vi "New Project.vi"(8 "error in (no error)":errorcluster, 11 "Editor.lvclass in":refnum<data-value>) -> (0 "error out":errorcluster, 2 "Cancelled":bool caption="cancelled", 3 "Editor.lvclass out":refnum<data-value>)   [LabVIEW 2015, in "Editor.lvclass"]
uses:
  Editor.lvclass
  Project.lvclass
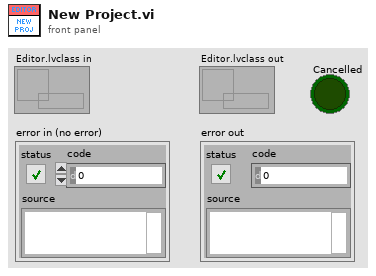
[diagram p1: front panel]
types:
  T1 = enum16{"Left Button", "Center Button", "Right Button", "Window Close"}
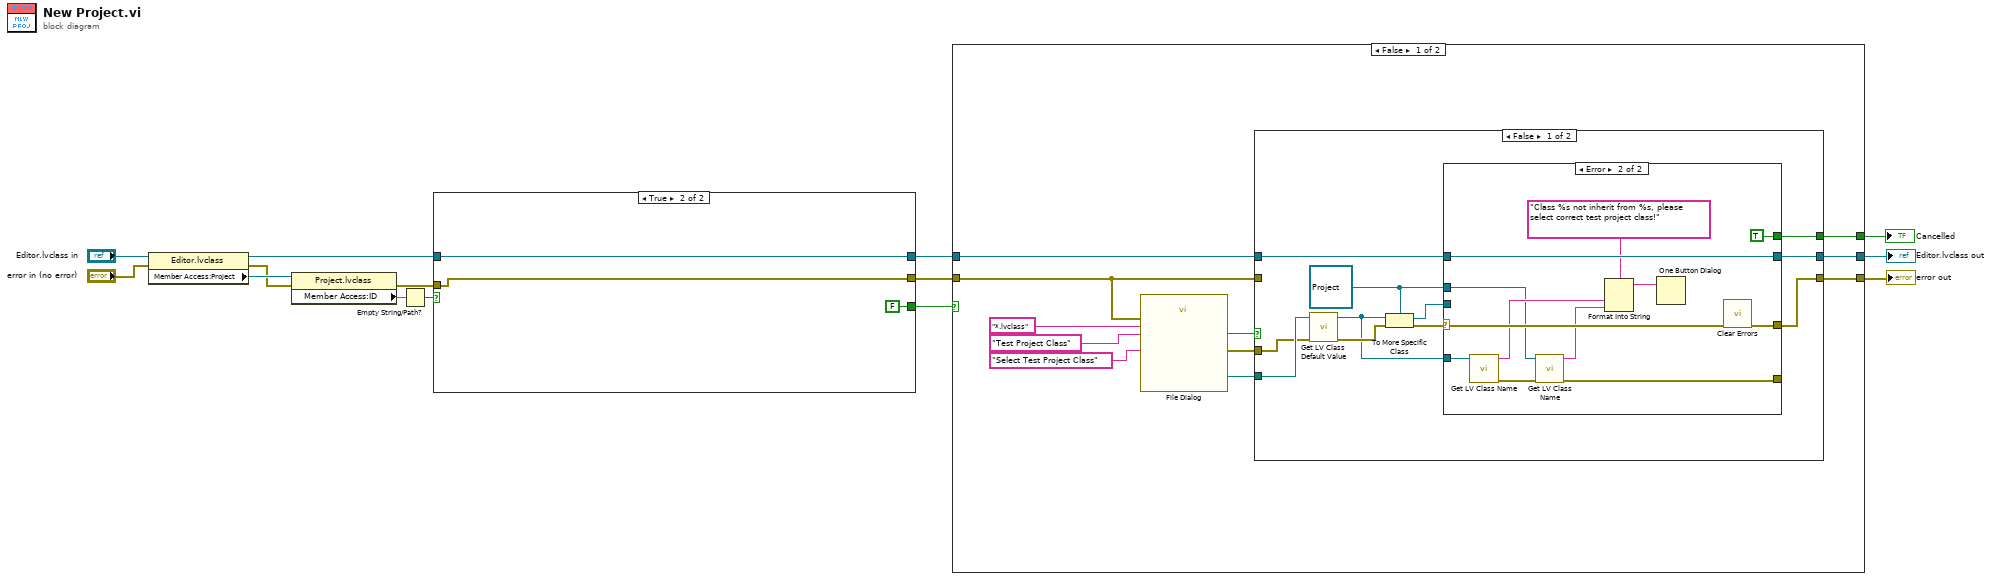
[diagram p0: block diagram]
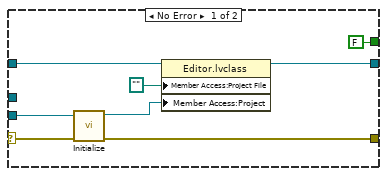
[diagram p2: hidden frame]
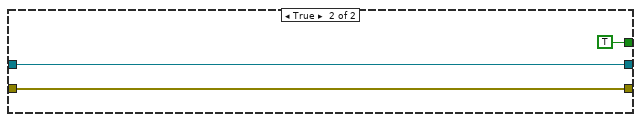
[diagram p3: hidden frame]
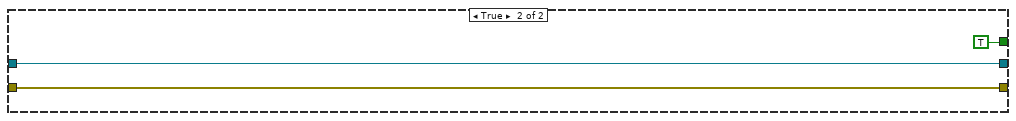
[diagram p4: hidden frame]
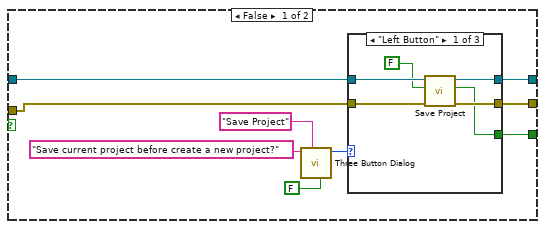
[diagram p5: hidden frame]
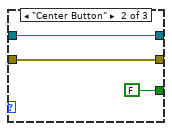
[diagram p6: hidden frame]
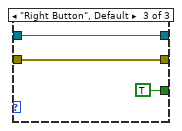
[diagram p7: hidden frame]
diagram:
  n1 = property class="Editor.lvclass"(reference="Editor.lvclass in", error in="error in (no error)") -> (reference out=w5:refnum<data-value>, error out=w7:errorcluster, "Member Access:Project"=w9:refnum<class "Project.lvclass">)
  n2 = property class="Project.lvclass"(reference=w9, error in=w7) -> (error out=w4:errorcluster, "Member Access:ID"=w8:string)  [unwired: 1 out]
  n3 = Empty String/Path?(string/path=w8) -> (empty?=w6:bool)
  n4 = case shown="True" w6 {
    tunnel: w5 -> [w19 w38]
    tunnel: w4 -> [w18 w37]
    tunnel: [w17 w38] -> w1
    tunnel: [w16 w37] -> w3
    tunnel: [w15 FALSE] -> w2
    frame False {
      n5 = call <vilib>:"Three Button Dialog.vi"("Allow user to close window? (TRUE)"=FALSE, "Window Title (\"\")"="Save Project" ("Window Title (\"\")"), "message"="Save current project before create a new project?") -> ("Which Button?"=w20:T1)  [unwired: 8 in]
      n6 = case shown="\"Left Button\"" w20 {
        tunnel: w19 -> [w29 w32 w35]
        tunnel: w18 -> [w27 w31 w34]
        tunnel: [w26 w32 w35] -> w17
        tunnel: [w25 w31 w34] -> w16
        tunnel: [w24 FALSE TRUE] -> w15
        frame "Left Button" {
          n7 = call "Save Project.vi"("error in (no error)"=w27, "Save As"=FALSE, "Editor.lvclass in"=w29) -> ("error out"=w25:errorcluster, "Cancelled"=w24:bool, "Editor.lvclass out"=w26:refnum<data-value>)  [unwired: 6 in]
        }
        frame "Center Button" {
        }
        frame "Right Button", Default {
        }
      }
    }
    frame True {
    }
  }
  n8 = case shown="False" w2 {
    tunnel: [w49 w86] -> w14
    tunnel: [w48 w85] -> w13
    tunnel: [w41 TRUE] -> w12
    tunnel: w1 -> [w40 w86]
    tunnel: w3 -> [w39 w85]
    frame False {
      n9 = call "File Dialog"("prompt"="Select Test Project Class" ("pattern (all files)"), "error in"=w39, "pattern (all files)"="*.lvclass", "pattern label"="Test Project Class" ("pattern (all files)")) -> ("selected path"=w44:path, "cancelled"=w42:bool, "error out"=w43:errorcluster)  [unwired: 8 in, 1 out]
      n10 = case shown="False" w42 {
        tunnel: [w60 w83] -> w49
        tunnel: w40 -> [w59 w83]
        tunnel: [w58 w81] -> w48
        tunnel: w44 -> [w55 _]
        tunnel: w43 -> [w50 _]
        tunnel: [w53 TRUE] -> w41
        tunnel: w39 -> [_ w81]
        frame False {
          w51 = refnum<class "Project.lvclass"> refnum ("Project.lvclass")
          n11 = call <vilib>:"Get LV Class Default Value.vi"("error in (no error)"=w50, "class path"=w55) -> ("error out"=w57:errorcluster, "object"=w52:refnum<class>)  [unwired: 8 in]
          n12 = To More Specific Class(target class=w51, reference=w52, error in=w57) -> (specific class reference=w56:refnum<class "Project.lvclass">, error out=w54:errorcluster)
          n13 = case shown="Error" w54 {
            selector: w54 -> [w62 w77]
            tunnel: [w66 w79] -> w60
            tunnel: w59 -> [w65 w79]
            tunnel: [w64 w78] -> w58
            tunnel: w56 -> [w63 _]
            tunnel: [FALSE TRUE] -> w53
            tunnel: w52 -> [_ w74]
            tunnel: w51 -> [_ w72]
            tunnel: [_ w70] -> _
            frame No Error {
              n14 = call-dynamic "Initialize.vi"("error in (no error)"=w62, "ProjectBase in"=w63) -> ("error out"=w64:errorcluster, "ProjectBase out"=w67:refnum<class "Project.lvclass">)  [unwired: 8 in]
              n15 = property class="Editor.lvclass"(reference=w65, "Member Access:Project File"=path "", "Member Access:Project"=w67) -> (reference out=w66:refnum<data-value>)  [unwired: 1 in, 1 out]
            }
            frame Error {
              n16 = call <vilib>:"Get LV Class Name.vi"("object"=w74) -> ("error out"=w75:errorcluster, "class name"=w73:string)  [unwired: 9 in]
              n17 = call <vilib>:"Get LV Class Name.vi"("error in (no error)"=w75, "object"=w72) -> ("error out"=w70:errorcluster, "class name"=w71:string)  [unwired: 8 in]
              n18 = Format Into String(format string="Class %s not inherit from %s, please select correct test project class!", w73, w71) -> (resulting string=w69:string)  [unwired: 2 in, 1 out]
              n19 = One Button Dialog(message=w69) -> ()  [unwired: 1 in, 1 out]
              n20 = call <vilib>:"Clear Errors.vi"("error in (no error)"=w77) -> ("error out"=w78:errorcluster)  [unwired: 5 in, 1 out]
            }
          }
        }
        frame True {
        }
      }
    }
    frame True {
    }
  }
  "Editor.lvclass out" <- w14
  "error out" <- w13
  "Cancelled" <- w12
